vi "SeCrTs-DC ON PPSU.vi"(8 "Error in":errorcluster) -> (0 "Fehler (Ausgang)":errorcluster caption="Error out")   [LabVIEW 2022 SP3]
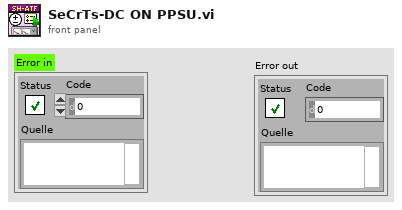
[diagram p1: front panel]
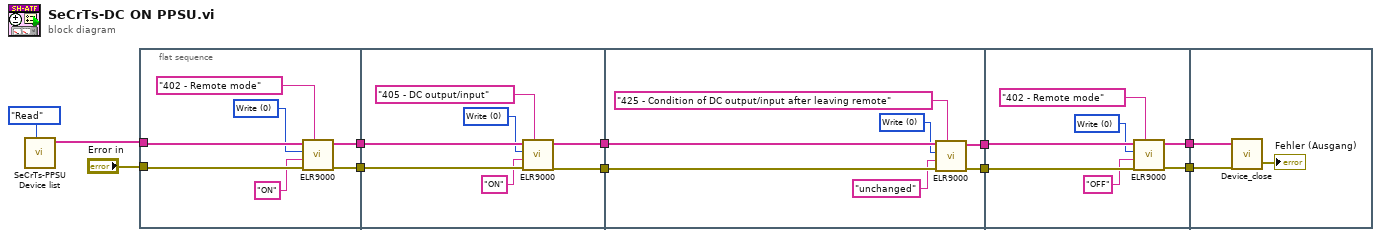
[diagram p0: block diagram]
diagram:
  n1 = call "SeCrTs-PPSU Device list.vi"("Enum"=enum16{"Read", "Write"}."Read") -> ("Device information arrayR"=w1:string[])  [unwired: 9 in, 1 out]
  n2 = flat-sequence {
    tunnel: "Error in" -> [w18]
    tunnel: w1 -> [w17]
    tunnel: [w13] -> w11
    tunnel: [w12] -> w10
    tunnel: w11 -> [w25]
    tunnel: w10 -> [w24]
    tunnel: [w20] -> w9
    tunnel: [w19] -> w8
    tunnel: w9 -> [w32]
    tunnel: w8 -> [w31]
    tunnel: [w27] -> w7
    tunnel: [w26] -> w6
    tunnel: w7 -> [w39]
    tunnel: w6 -> [w38]
    tunnel: [w34] -> w5
    tunnel: [w33] -> w4
    tunnel: w5 -> [w42]
    tunnel: w4 -> [w41]
    frame #0 {
      w15 = u8 0 items=["Write", "Read"] ("Access")
      n3 = call <instrlib>:"ELR9000.vi"("Command list"="402 - Remote mode", "Error in"=w18, "Value"="ON", "Access"=w15, "Device information in"=w17) -> ("Error out"=w12:errorcluster, "Device information out"=w13:string[])  [unwired: 1 in, 2 out]
    }
    frame #1 {
      w22 = u8 0 items=["Write", "Read"] ("Access")
      n4 = call <instrlib>:"ELR9000.vi"("Command list"="405 - DC output/input", "Error in"=w24, "Value"="ON", "Access"=w22, "Device information in"=w25) -> ("Error out"=w20:errorcluster, "Device information out"=w19:string[])  [unwired: 1 in, 2 out]
    }
    frame #2 {
      w30 = u8 0 items=["Write", "Read"] ("Access")
      n5 = call <instrlib>:"ELR9000.vi"("Command list"="425 - Condition of DC output/input after leaving remote", "Error in"=w32, "Value"="unchanged", "Access"=w30, "Device information in"=w31) -> ("Error out"=w27:errorcluster, "Device information out"=w26:string[])  [unwired: 1 in, 2 out]
    }
    frame #3 {
      w36 = u8 0 items=["Write", "Read"] ("Access")
      n6 = call <instrlib>:"ELR9000.vi"("Command list"="402 - Remote mode", "Error in"=w39, "Value"="OFF", "Access"=w36, "Device information in"=w38) -> ("Error out"=w34:errorcluster, "Device information out"=w33:string[])  [unwired: 1 in, 2 out]
    }
    frame #4 {
      n7 = call <instrlib>:"Device_close.vi"("error in (no error)"=w42, "Device information in"=w41) -> ("Fehler (Ausgang)"=→"Fehler (Ausgang)":errorcluster)  [unwired: 3 in]
    }
  }
